vi "RS 485 COM Out.vi"(11 "Port":T1=enum."None") -> (3 "9871 COM":T2={"Data"=[0, 0, 0, 0, 0, 0, 0, 0, 0, 0, 0, 0, 0, 0, 0, 0, 0, 0, 0, 0, 0, 0, 0, 0, 0, 0, 0, 0, 0, 0], "NumBytes"=0, "Port"=enum."Port 1", "Wait for Reply"=FALSE})   [LabVIEW 2015]
uses:
  <vilib>/eio/EIOMethodNode/EIOMethodNode.xnode
  <vilib>/rvi/eio/common/nirviEmuTemplateMethod_errors.vi
  Port Selector.ctl
  9871 COM In.ctl
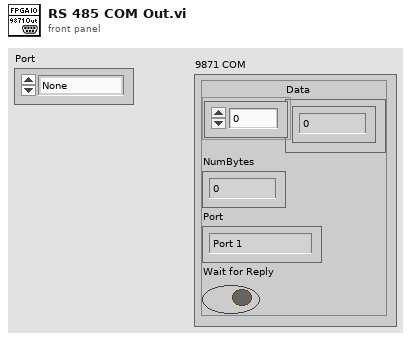
[diagram p1: front panel]
types:
  T1 = typedef "Port Selector.ctl" = enum16{"Port 1", "Port 2", "Port 3", "Port 4", "None"}
  T2 = typedef "9871 COM In.ctl" = cluster{"Data":u8[], "NumBytes":i32, "Port":T1, "Wait for Reply":bool}
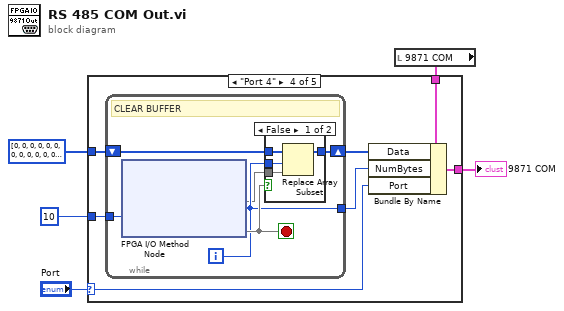
[diagram p0: block diagram]
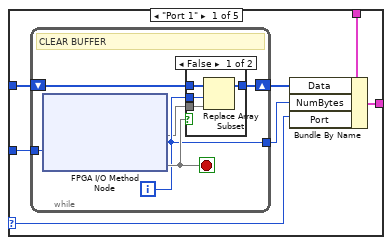
[diagram p2: hidden frame]
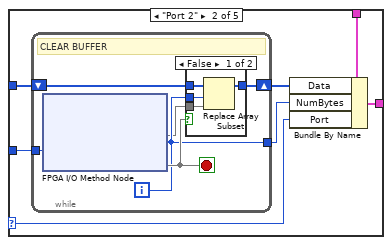
[diagram p4: hidden frame]
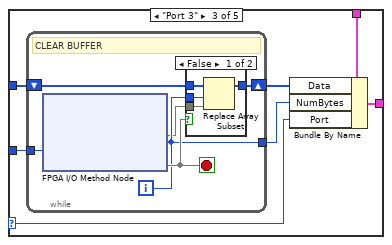
[diagram p6: hidden frame]
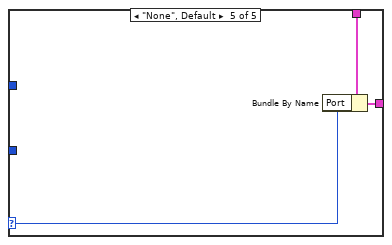
[diagram p9: hidden frame]
diagram:
  n1 = local read "9871 COM"() -> (w2:T2)
  n2 = case shown="\"Port 4\"" "Port" {
    selector: "Port" -> [w9 w28 w46 w64 w79]
    tunnel: [w12 w27 w45 w63 w78] -> w5
    tunnel: u8[] [0, 0, 0, 0, 0, 0, 0, 0, 0, 0, 0, 0, 0, 0, 0, 0, 0, 0, 0, 0, 0, 0, 0, 0, 0, 0, 0, 0, 0, 0] -> [w8 w26 w44 w62 _]
    tunnel: w2 -> [w7 w25 w43 w61 w80]
    tunnel: 10 ("Timeout (ms)") -> [w6 w24 w42 w60 _]
    frame "Port 1" {
      n3 = while {
        shift-right: [w17] -> w11
        shift-left: w8 -> [w18]
        tunnel: [w15] -> w10
        tunnel: w6 -> [w13]
        i -> [w15]
        stop <- w16 stop-if-true
        # "CLEAR BUFFER"
        n4 = xnode "FPGA I/O Method Node"("Timeout (ms)"=w13) -> ("Data"=w14, "Timed Out"=w16)  [unwired: 1 in, 1 out]
        n5 = case shown="False" w16 {
          tunnel: w18 -> [w22 w23]
          tunnel: [w19 w23] -> w17
          tunnel: w14 -> [w21 _]
          tunnel: w15 -> [w20 _]
          frame False {
            n6 = Replace Array Subset(array=w22, new element=w21, index=w20) -> (w19:u8[])
          }
          frame True {
          }
        }
      }
      n7 = Bundle By Name(cluster=w7, "Data"=w11, "NumBytes"=w10, "Port"=w9) -> (w12:T2)
    }
    frame "Port 2" {
      n8 = while {
        shift-right: [w35] -> w30
        shift-left: w26 -> [w36]
        tunnel: [w33] -> w29
        tunnel: w24 -> [w31]
        i -> [w33]
        stop <- w34 stop-if-true
        # "CLEAR BUFFER"
        n9 = xnode "FPGA I/O Method Node"("Timeout (ms)"=w31) -> ("Data"=w32, "Timed Out"=w34)  [unwired: 1 in, 1 out]
        n10 = case shown="False" w34 {
          tunnel: w36 -> [w40 w41]
          tunnel: [w37 w41] -> w35
          tunnel: w32 -> [w39 _]
          tunnel: w33 -> [w38 _]
          frame False {
            n11 = Replace Array Subset(array=w40, new element=w39, index=w38) -> (w37:u8[])
          }
          frame True {
          }
        }
      }
      n12 = Bundle By Name(cluster=w25, "Data"=w30, "NumBytes"=w29, "Port"=w28) -> (w27:T2)
    }
    frame "Port 3" {
      n13 = while {
        shift-right: [w53] -> w48
        shift-left: w44 -> [w54]
        tunnel: [w51] -> w47
        tunnel: w42 -> [w49]
        i -> [w51]
        stop <- w52 stop-if-true
        # "CLEAR BUFFER"
        n14 = xnode "FPGA I/O Method Node"("Timeout (ms)"=w49) -> ("Data"=w50, "Timed Out"=w52)  [unwired: 1 in, 1 out]
        n15 = case shown="False" w52 {
          tunnel: w54 -> [w58 w59]
          tunnel: [w55 w59] -> w53
          tunnel: w50 -> [w57 _]
          tunnel: w51 -> [w56 _]
          frame False {
            n16 = Replace Array Subset(array=w58, new element=w57, index=w56) -> (w55:u8[])
          }
          frame True {
          }
        }
      }
      n17 = Bundle By Name(cluster=w43, "Data"=w48, "NumBytes"=w47, "Port"=w46) -> (w45:T2)
    }
    frame "Port 4" {
      n18 = while {
        shift-right: [w71] -> w66
        shift-left: w62 -> [w72]
        tunnel: [w69] -> w65
        tunnel: w60 -> [w67]
        i -> [w69]
        stop <- w70 stop-if-true
        # "CLEAR BUFFER"
        n19 = xnode "FPGA I/O Method Node"("Timeout (ms)"=w67) -> ("Data"=w68, "Timed Out"=w70)  [unwired: 1 in, 1 out]
        n20 = case shown="False" w70 {
          tunnel: w72 -> [w76 w77]
          tunnel: [w73 w77] -> w71
          tunnel: w68 -> [w75 _]
          tunnel: w69 -> [w74 _]
          frame False {
            n21 = Replace Array Subset(array=w76, new element=w75, index=w74) -> (w73:u8[])
          }
          frame True {
          }
        }
      }
      n22 = Bundle By Name(cluster=w61, "Data"=w66, "NumBytes"=w65, "Port"=w64) -> (w63:T2)
    }
    frame "None", Default {
      n23 = Bundle By Name(cluster=w80, "Port"=w79) -> (w78:T2)
    }
  }
  "9871 COM" <- w5
